vi "MSFET202_pH_CalibCalc.vi"(1 "Eint":dbl=1.679301629734707) -> (0 "pHint":dbl=8.77599208192754)   [LabVIEW 2018]
panel:
  in  "calpH":dbl=7.0
  in  "calEint":dbl=1.37533
  # "pH Calibration & Calculation (MSFET3332 202)"
  # "INPUTS"
  # "<-- Automatically inputed"
  # "OUTPUT"
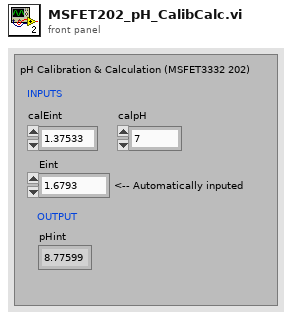
[diagram p1: front panel]
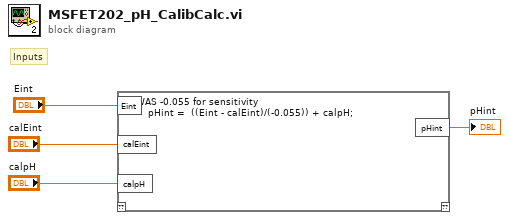
[diagram p0: block diagram]
diagram:
  # "Inputs"
  n1 = script code="%WAS -0.055 for sensitivity\n       pHint =  ((Eint - calEint)/(-0.055)) + calpH;"("calEint"="calEint", "calpH"="calpH", "Eint"="Eint") -> ("pHint"=→"pHint":dbl)  [unwired: 1 in, 1 out]
